vi "Run Service.vi"(11 "MeasurementLink Server User Events":T1) -> (0 "error out":errorcluster)   [LabVIEW 2021, in "Service.lvlib"]
uses:
  Service.lvlib
  <vilib>/Plug-In SDKs/Measurements/Helpers/TypeDefs/Measurement Server User Settings.ctl
  <vilib>/Plug-In SDKs/Measurements/Helpers/TypeDefs/Stop Server User Event.ctl
  <vilib>/Plug-In SDKs/Measurements/Helpers/TypeDefs/Measurement Service Version.ctl
  Advanced/MeasurementPlugin.lvclass
  C:/Program Files/National Instruments/LabVIEW 2021/vi.lib/Plug-In SDKs/Measurements/Measurement Plugin Service/Measurement Plugin Service.lvclass
  <vilib>/Plug-In SDKs/Measurements/NI Measurement Plug-In SDK.lvlib
panel:
  # "Run this VI to start the measurement service.  A window will appear that provides basic information about the running service.\n\nUse the stop button on the window that appears to stop the measurement service."
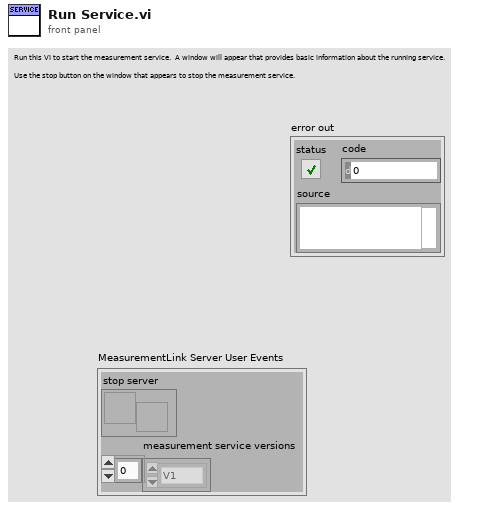
[diagram p1: front panel]
types:
  T1 = typedef "NI Measurement Plug-In SDK.lvlib/Measurement Server User Settings.ctl" = cluster{"stop server":T2, "measurement service versions":T3[]}
  T2 = typedef "NI Measurement Plug-In SDK.lvlib/Stop Server User Event.ctl" = refnum<user-event>
  T3 = typedef "NI Measurement Plug-In SDK.lvlib/Measurement Service Version.ctl" = enum16{"V1", "V2"}
  T4 = enum32{"Invalid", "Standard", "Closed", "Hidden", "Minimized", "Maximized"}
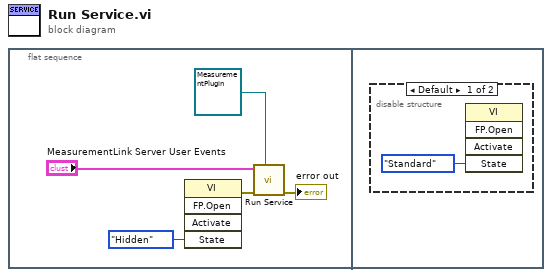
[diagram p0: block diagram]
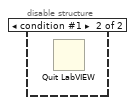
[diagram p2: hidden frame]
diagram:
  n1 = flat-sequence {
    frame #0 {
      n2 = invoke class="VI" method="FP.Open"("State"=T4."Hidden") -> (error out=w3:errorcluster)  [unwired: 4 in, 4 out]
      n3 = call <vilib>:"Run Service.vi"("measurement"=refnum<class "MeasurementPlugin.lvclass"> refnum ("MeasurementLink Measurement Template.lvlib:Measurement Customizations.lvclass"), "error in"=w3, "measurementlink server user settings"="MeasurementLink Server User Events") -> ("error out"=→"error out":errorcluster)  [unwired: 8 in]
    }
    frame #1 {
      n4 = disable-structure shown="Default" {
        frame condition #0 (active) {
          n5 = invoke class="VI" method="FP.Open"("State"=T4."Standard") -> ()  [unwired: 4 in, 5 out]
        }
        frame condition #1 {
          n6 = Quit LabVIEW() -> ()  [unwired: 1 in]
        }
      }
    }
  }
